vi "GT_BufMove.vi"(4 "modal":i16, 5 "acc":dbl, 6 "vel":dbl, 7 "pos":i32, 8 "fifo":i16, 9 "MoveAxis in":T1=1 items=["Axis Control"=0, "Axis 1"=1, "Axis 2"=2, "Axis 3"=3, "Axis 4"=4, "Axis 5"=5, "Axis 6"=6, "Axis 7"=7, "Axis 8"=8, "Vector Space Control"=16, "Vector Space 1"=17, "Vector Space 2"=18, "Vector Space 3"=19, "Vector Space 4"=20], 10 "crd":i16, 11 "rtn_In":cluster{"rtn":i16, "Func":string}) -> (0 "fifo out":i16, 1 "crd out":i16, 2 "MoveAxis out":T1=1 items=["Axis Control"=0, "Axis 1"=1, "Axis 2"=2, "Axis 3"=3, "Axis 4"=4, "Axis 5"=5, "Axis 6"=6, "Axis 7"=7, "Axis 8"=8, "Vector Space Control"=16, "Vector Space 1"=17, "Vector Space 2"=18, "Vector Space 3"=19, "Vector Space 4"=20], 3 "rtn_Out":cluster{"rtn":i16, "Func":string})   [LabVIEW 2014]
uses:
  <vilib>/Motion/FlexMotion/CustomControls/CustomControls.llb/AxisOrVectorSpaceControl To Control.flx
  VC6/gts.dll
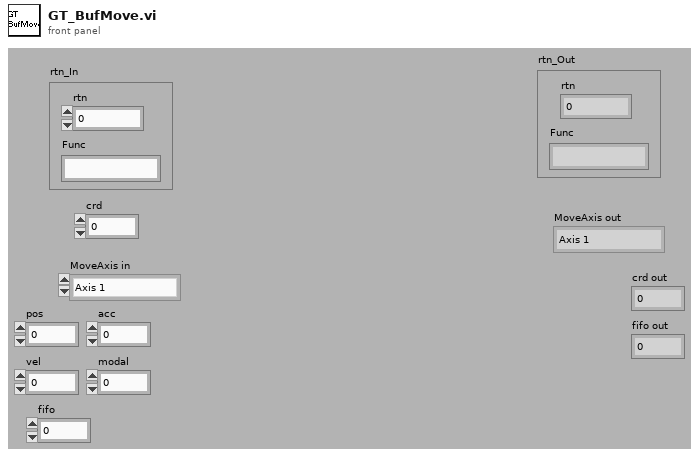
[diagram p1: front panel]
types:
  T1 = typedef "AxisOrVectorSpaceControl To Control.flx" = u16
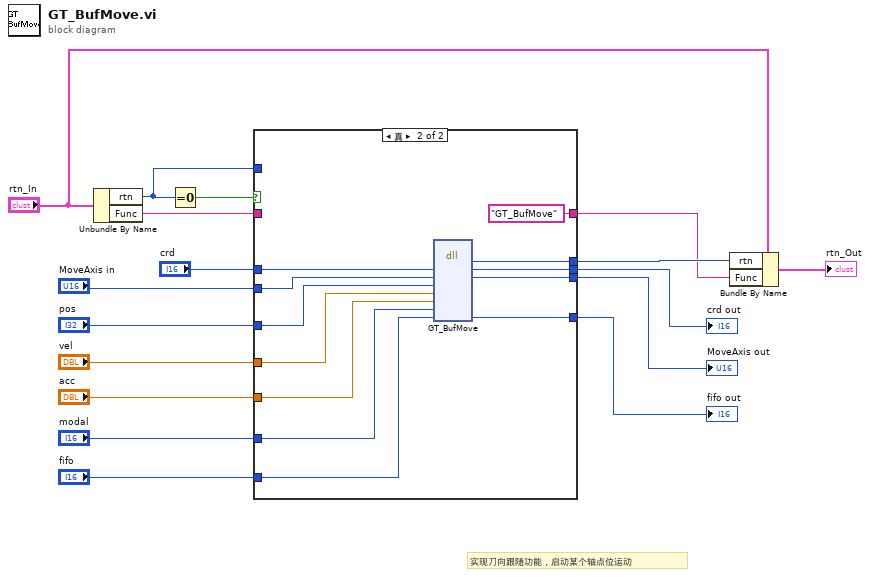
[diagram p0: block diagram]
diagram:
  # "实现刀向跟随功能，启动某个轴点位运动"
  n1 = Unbundle By Name("rtn_In") -> ("rtn"=w5:i16, "Func"=w4:string)
  n2 = Equal To 0?(x=w5) -> (x = 0?=w17:bool)
  n3 = case shown="真" w17 {
    tunnel: [w22 w34] -> w14
    tunnel: "crd" -> [w19 w33]
    tunnel: "MoveAxis in" -> [w18 w32]
    tunnel: "pos" -> [_ w31]
    tunnel: "vel" -> [_ w30]
    tunnel: "acc" -> [_ w29]
    tunnel: "modal" -> [_ w28]
    tunnel: "fifo" -> [w20 w27]
    tunnel: [w19 w26] -> w7
    tunnel: [w18 w25] -> w1
    tunnel: [w20 w24] -> w6
    tunnel: w5 -> [w22 _]
    tunnel: w4 -> [w21 _]
    tunnel: [w21 "GT_BufMove" ("Func")] -> w3
    frame False {
    }
    frame True {
      n4 = dll-call lib="PTH2Fabs DNewGTS AC-800LWin7版源程序-20170926gts85VC6gts.dll" fn="GT_BufMove"("crd"=w33, "moveAxis"=w32, "pos"=w31, "vel"=w30, "acc"=w29, "modal"=w28, "fifo"=w27) -> ("rtn"=w34:i16, "crd"=w26:i16, "moveAxis"=w25:i16, "fifo"=w24:i16)  [unwired: 7 in, 2 out]
    }
  }
  "crd out" <- w7
  "fifo out" <- w6
  "MoveAxis out" <- w1
  n5 = Bundle By Name(cluster="rtn_In", "rtn"=w14, "Func"=w3) -> (→"rtn_Out":cluster{"rtn":i16, "Func":string})
